vi "main.vi"(1 "chessboard_size":u8=8, 2 "starting_square":T1) -> ()   [LabVIEW 2020, in "core.lvlib"]
uses:
  core.lvlib
  core_data/chess_square--chess notation.ctl
  core_data/file--enum.ctl
  core_data/rank--enum.ctl
  action.ctl
  check_has_tour_been_found.vi
  check_has_unreacheable_square_been_formed.vi
  check_any_corner_islands.vi
  convert--duration to formatted string.vi
  get_chessboard_square.vi
  check_island.vi
  check_head_is_neighbour.vi
  get all unexplored neighbours.vi
  pause (global variable).vi
  core_data/library_variable.vi
  pause after every move (global variable).vi
  main/Enqueue--button_press_pause.vi
  core_wait (global variable).vi
  convert--chessboard_index to chess_square (string).vi
  get tour type.vi
  core_data/chessboard_index.ctl
  core_data/completed_tour.ctl
  core_data/tour type (enum).ctl
  core_data/core_data.lvlib
  core_data/tour_in_progress.ctl
  core_data/core_data.ctl
  core_data/neighbour_square.ctl
  core_data/chess_square.ctl
  global_stop_flag/global_stop_flag.lvlib
  main/main.lvlib
  PTRL/timing_utilities/timing_utilities.lvlib
  PTRL/dev_and_debug_tools/dev_and_debug_tools.lvlib
panel:
  out "complete_tour indexes":i32[](array[numeric])
  out "States out (index 0 = oldest)":string[](array[string])
  out "iteration":i32
  # "Core"
  # "Development\ncontrols/indicators useful for development and testing, but which are not outputs of the VI"
  # "Input\nInputs to the VI"
  # "Output\nOutputs of the VI"
  # "Description\n\nBlank VI with error handling case. \n\nSummarize the use of this VI in this space."
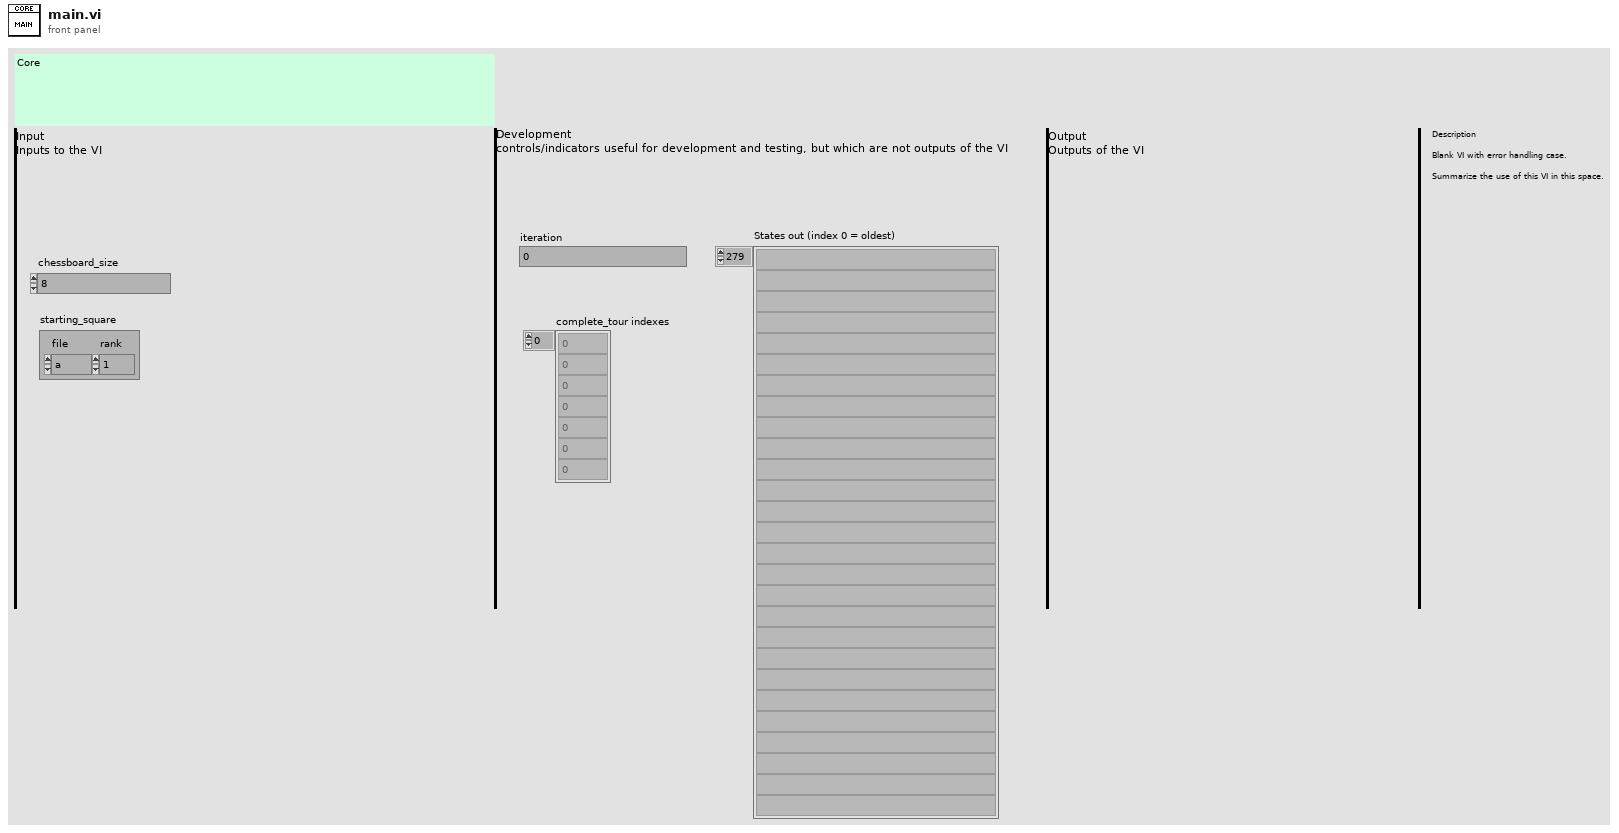
[diagram p1: front panel]
types:
  T1 = typedef "core.lvlib/core_data.lvlib/chess_square--chess notation.ctl" = cluster{"file":T2, "rank":T3}
  T2 = typedef "core.lvlib/core_data.lvlib/file--enum.ctl" = enum16{"a", "b", "c", "d", "e", "f", "g", "h"}
  T3 = typedef "core.lvlib/core_data.lvlib/rank--enum.ctl" = enum16{"1", "2", "3", "4", "5", "6", "7", "8"}
  T4 = typedef "core.lvlib/action.ctl" = enum16{"init", "move_forward", "move_backward", "complete_tour", "exit", "be idle (do nothing)"}
  T5 = typedef "core.lvlib/core_data.lvlib/chessboard_index.ctl" = cluster{"row":u8, "column":u8}
  T6 = typedef "core.lvlib/core_data.lvlib/core_data.ctl" = cluster{"tour_in_progress":T7, "total no. of moves forward":u64, "total no. of moves backward":u64, "chessboard":T8[][], "square_to_move_forward_to":T5}
  T7 = typedef "core.lvlib/core_data.lvlib/tour_in_progress.ctl" = cluster{"start_time":timestamp, "tour":T5[], "no. of moves forward":u64, "no. of moves backward":u64}
  T8 = typedef "core.lvlib/core_data.lvlib/chess_square.ctl" = cluster{"Explored?":bool, "neighbouring_squares":T9[]}
  T9 = typedef "core.lvlib/core_data.lvlib/neighbour_square.ctl" = cluster{"row":u8, "column":u8, "exhausted?":bool}
  T10 = typedef "core.lvlib/core_data.lvlib/completed_tour.ctl" = cluster{"complete_tour":T5[], "start square":string, "end square":string, "tour type":T11, "start_time":timestamp, "end_time":timestamp, "duration (seconds)":dbl, "duration (formatted string)":string, "no. of moves forward":u64, "no. of moves backward":u64, "total no. of moves since core started running":u64}
  T11 = typedef "core.lvlib/core_data.lvlib/tour type (enum).ctl" = enum16{"open", "closed"}
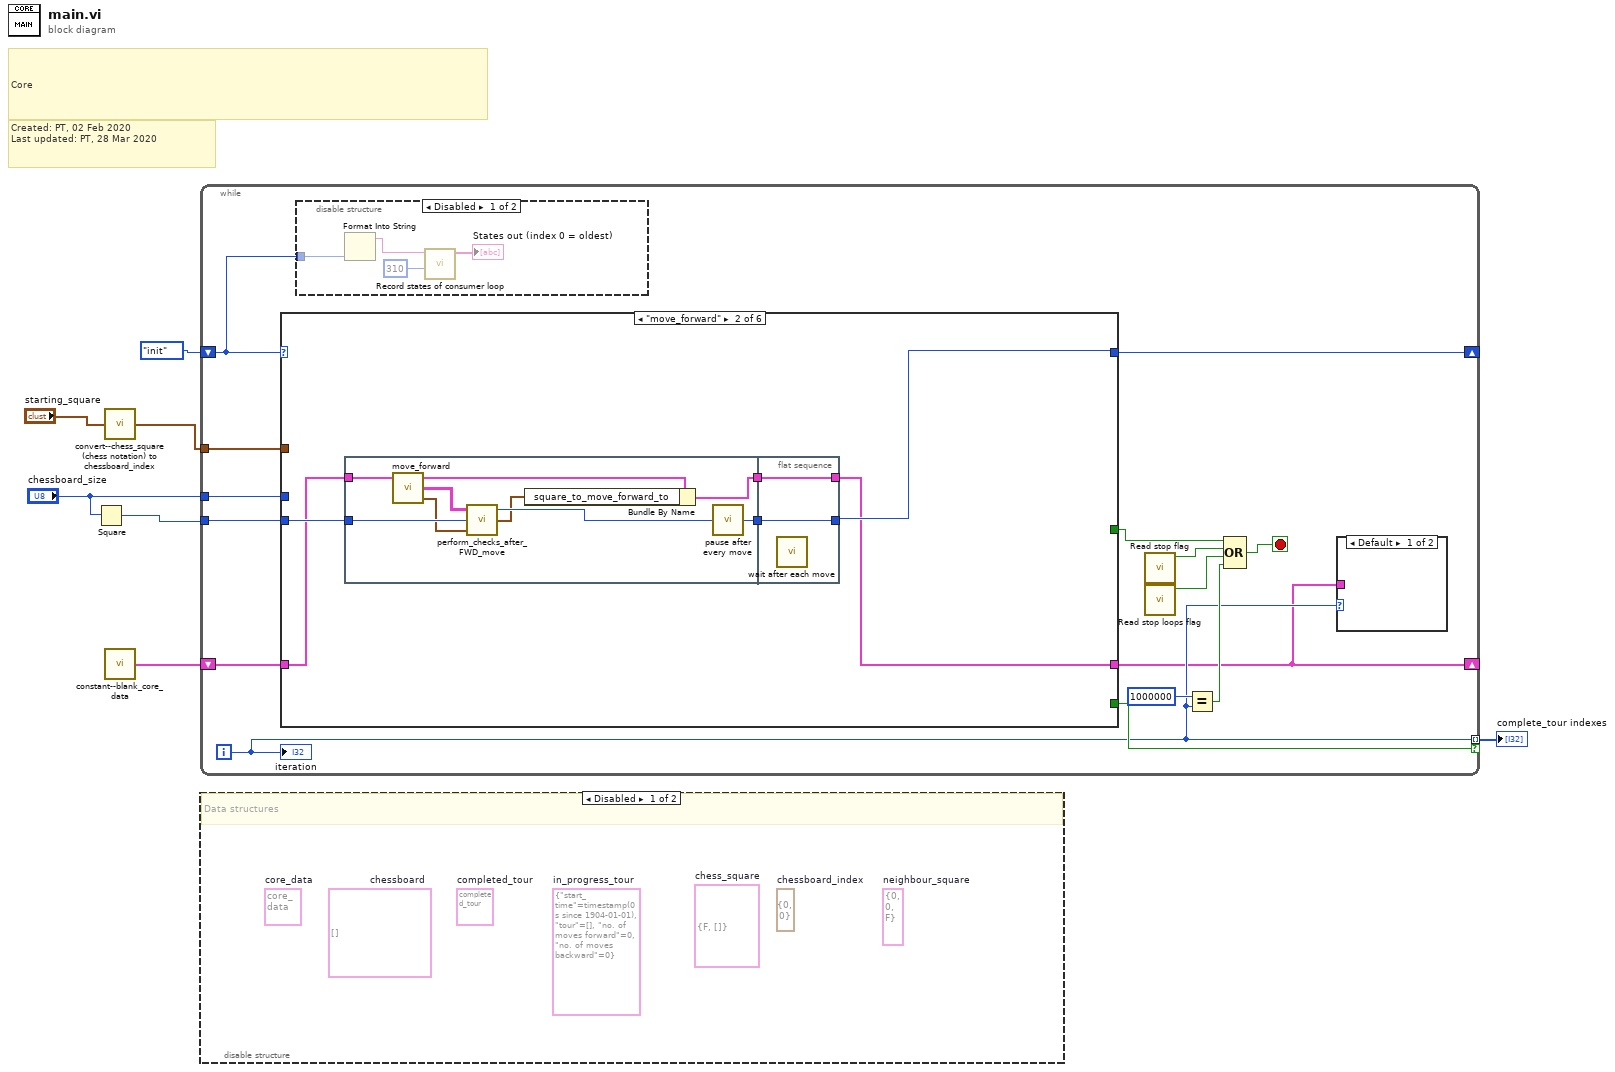
[diagram p0: block diagram]
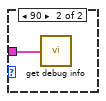
[diagram p3: hidden frame]
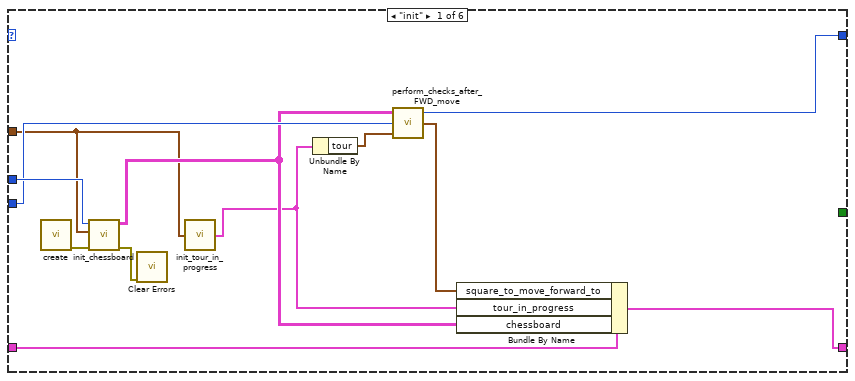
[diagram p4: hidden frame]
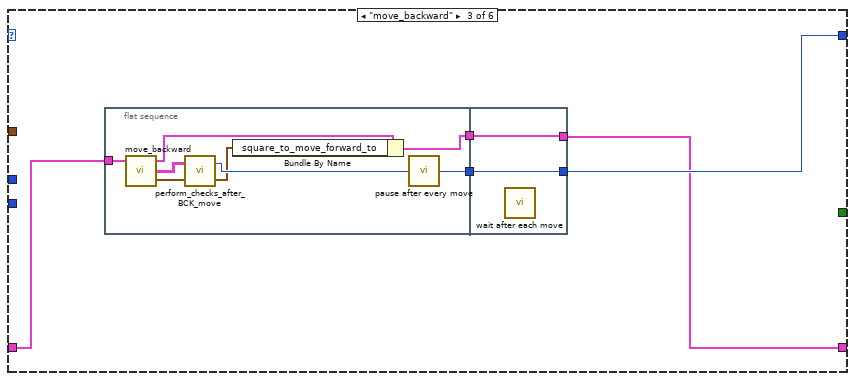
[diagram p5: hidden frame]
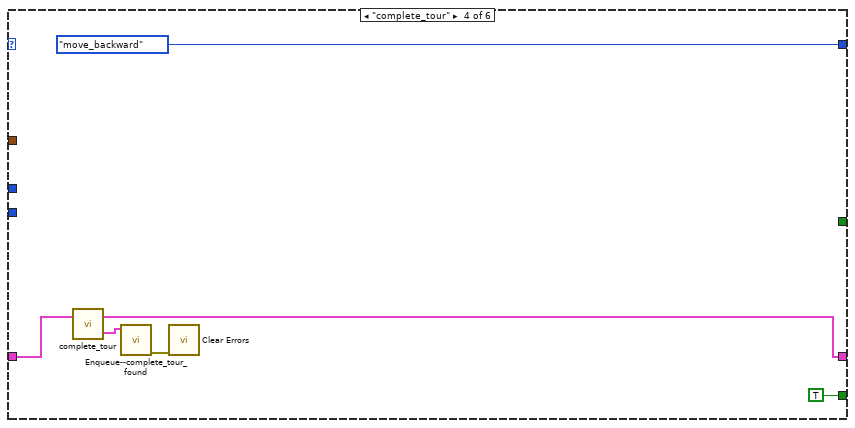
[diagram p6: hidden frame]
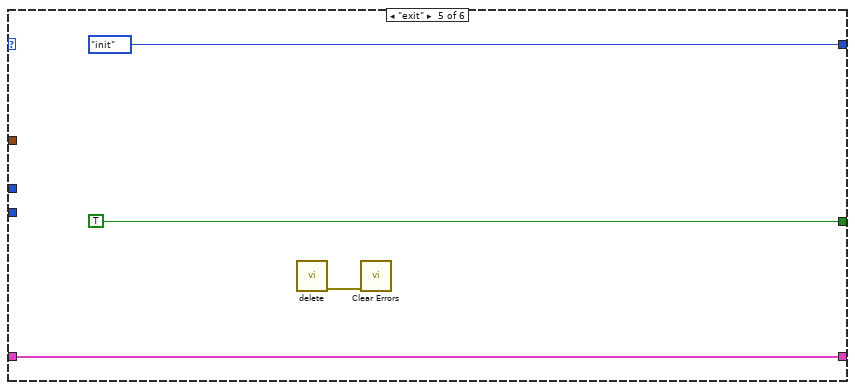
[diagram p7: hidden frame]
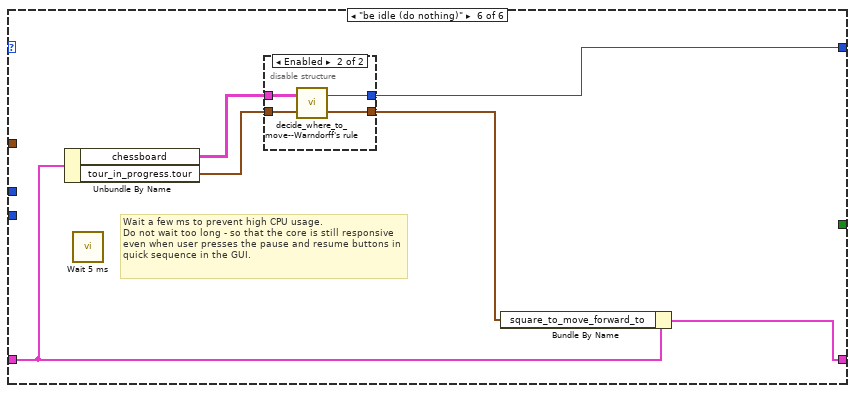
[diagram p8: hidden frame]
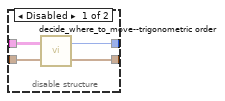
[diagram p9: hidden frame]
diagram:
  # "Core"
  # "Created: PT, 02 Feb 2020\nLast updated: PT, 28 Mar 2020"
  n1 = Square(x="chessboard_size") -> (x^2=w5:u8)
  n2 = call "convert--chess_square (chess notation) to chessboard_index.vi"("chess_square (chess notation)"="starting_square") -> ("chessboard_index"=w3:T5)
  n3 = call "constant--blank_core_data.vi"() -> ("blank core_data"=w2:T6)
  n4 = while {
    shift-right: [w22] -> _
    shift-left: action."init" ("action (default = init)") -> [w13]
    tunnel: w3 -> [w21]
    tunnel: "chessboard_size" -> [w20]
    tunnel: w5 -> [w15]
    shift-right: [w8] -> _
    shift-left: w2 -> [w14]
    tunnel: [w9] -> w1 mode=indexing if=w10
    i -> [w9]
    stop <- w18 stop-if-true
    n5 = case shown="\"move_forward\"" w13 {
      tunnel: [w36 w45 w60 action."move_backward" ("action") action."init" ("action") w87] -> w22
      tunnel: w21 -> [w34 _ _ _ _ _]
      tunnel: w20 -> [w39 _ _ _ _ _]
      tunnel: w15 -> [w37 w43 _ _ _ _]
      tunnel: [_ _ _ _ TRUE _] -> w19
      tunnel: w14 -> [w32 w42 w59 w74 w79 w83]
      tunnel: [w30 w40 w57 w73 w79 w84] -> w8
      tunnel: [_ _ _ TRUE _ _] -> w10
      frame "init" {
        n6 = call "create.vi"() -> ("error out"=w38:errorcluster)  [unwired: 11 in]
        n7 = call "init_chessboard.vi"("error in (no error)"=w38, "starting_square"=w34, "chessboard_size"=w39) -> ("error out"=w33:errorcluster, "chessboard (populated)"=w35:T8[][])  [unwired: 7 in]
        n8 = call <vilib>:"Clear Errors.vi"("error in (no error)"=w33) -> ()  [unwired: 5 in, 2 out]
        n9 = call "init_tour_in_progress.vi"("starting_square"=w34) -> ("blank_tour_in_progress"=w28:T7)
        n10 = Unbundle By Name(w28) -> ("tour"=w31:T5[])
        n11 = call "perform_checks_after_FWD_move.vi"("tour_in_progress"=w31, "no. of squares on chessboard"=w37, "chessboard"=w35) -> ("square_to_move_forward_to"=w29:T5, "next action"=w36:T4)  [unwired: 1 in]
        n12 = Bundle By Name(cluster=w32, "square_to_move_forward_to"=w29, "tour_in_progress"=w28, "chessboard"=w35) -> (w30:T6)
      }
      frame "move_forward" {
        n13 = flat-sequence {
          tunnel: [w53] -> w44
          tunnel: w43 -> [w51]
          tunnel: w42 -> [w49]
          tunnel: [w47] -> w41
          tunnel: [w56] -> w45
          tunnel: w44 -> [w56]
          tunnel: [w55] -> w40
          tunnel: w41 -> [w55]
          frame #0 {
            n14 = call "move_forward.vi"("core_data in"=w49) -> ("tour in progress"=w50:T5[], "chessboard"=w52:T8[][], "core_data out"=w48:T6)  [unwired: 2 in]
            n15 = call "perform_checks_after_FWD_move.vi"("tour_in_progress"=w50, "no. of squares on chessboard"=w51, "chessboard"=w52) -> ("square_to_move_forward_to"=w46:T5, "next action"=w54:T4)  [unwired: 1 in]
            n16 = Bundle By Name(cluster=w48, "square_to_move_forward_to"=w46) -> (w47:T6)
            n17 = call "pause after every move.vi"("next action in"=w54) -> ("next action out"=w53:T4)
          }
          frame #1 {
            n18 = call "wait after each move.vi"() -> ()  [unwired: 12 in]
          }
        }
      }
      frame "move_backward" {
        n19 = flat-sequence {
          tunnel: [w68] -> w61
          tunnel: w59 -> [w65]
          tunnel: [w63] -> w58
          tunnel: [w71] -> w60
          tunnel: w61 -> [w71]
          tunnel: [w70] -> w57
          tunnel: w58 -> [w70]
          frame #0 {
            n20 = call "move_backward.vi"("core_data in"=w65) -> ("tour in progress"=w66:T5[], "chessboard"=w67:T8[][], "core_data out"=w64:T6)  [unwired: 2 in]
            n21 = call "perform_checks_after_BCK_move.vi"("tour in progress"=w66, "chessboard"=w67) -> ("square_to_move_forward_to"=w62:T5, "next action"=w69:T4)
            n22 = Bundle By Name(cluster=w64, "square_to_move_forward_to"=w62) -> (w63:T6)
            n23 = call "pause after every move.vi"("next action in"=w69) -> ("next action out"=w68:T4)
          }
          frame #1 {
            n24 = call "wait after each move.vi"() -> ()  [unwired: 12 in]
          }
        }
      }
      frame "complete_tour" {
        n25 = call "complete_tour.vi"("core_data in"=w74) -> ("the recently completed tour"=w75:T10, "core_data out"=w73:T6)  [unwired: 1 in]
        n26 = call "Enqueue--complete_tour_found.vi"("completed_tour"=w75) -> ("error out"=w76:errorcluster)  [unwired: 10 in]
        n27 = call <vilib>:"Clear Errors.vi"("error in (no error)"=w76) -> ()  [unwired: 5 in, 2 out]
      }
      frame "exit" {
        n28 = call "delete.vi"() -> ("error out"=w78:errorcluster)  [unwired: 10 in, 1 out]
        n29 = call <vilib>:"Clear Errors.vi"("error in (no error)"=w78) -> ()  [unwired: 5 in, 2 out]
      }
      frame "be idle (do nothing)" {
        # "Wait a few ms to prevent high CPU usage.\nDo not wait too long - so that the core is still responsive even when user presses the pause and resume buttons in quick sequence in the GUI."
        n30 = Unbundle By Name(w83) -> ("chessboard"=w86:T8[][], "tour_in_progress.tour"=w85:T5[])
        n31 = call "Wait 5 ms.vi"() -> ()  [unwired: 11 in, 1 out]
        n32 = disable-structure shown="Enabled" {
          disable-tunnel: [w91 w92] -> w82
          disable-tunnel: [w90 w93] -> w87
          disable-tunnel: w86 -> [w89 w95]
          disable-tunnel: w85 -> [w88 w94]
          frame Disabled {
            n33 = call "decide_where_to_move--trigonometric order.vi"("tour_in_progress"=w88, "chessboard"=w89) -> ("square_to_move_forward_to"=w91:T5, "action"=w90:T4)
          }
          frame Enabled {
            n34 = call "decide_where_to_move--Warndorff's rule.vi"("tour_in_progress"=w94, "chessboard"=w95) -> ("square_to_move_forward_to"=w92:T5, "action"=w93:T4)
          }
        }
        n35 = Bundle By Name(cluster=w83, "square_to_move_forward_to"=w82) -> (w84:T6)
      }
    }
    n36 = disable-structure shown="Disabled" {
      disable-tunnel: w13 -> [w26 _]
      frame Disabled {
        n37 = Format Into String(w26) -> (resulting string=w25:string)  [unwired: 3 in, 1 out]
        n38 = call "Record states of consumer loop.vi"("n (dflt=100)"=u32 310, "State in"=w25) -> ("States out (index 0 = oldest)"=→"States out (index 0 = oldest)":string[])  [unwired: 7 in, 2 out]
      }
      frame Enabled {
      }
    }
    n39 = call "Read stop flag.vi"() -> ("Stop core?"=w17:bool)  [unwired: 10 in, 1 out]
    n40 = call "Read stop loops flag.vi"() -> ("Stop all loops?"=w16:bool)  [unwired: 10 in, 1 out]
    n41 = Equal?(x=1000000, y=w9) -> (x = y?=w12:bool)
    n42 = Compound Arithmetic op=OR(w19, w17, w16, w12) -> (w18:bool)
    n43 = case shown="Default" w9 {
      tunnel: w8 -> [_ w27]
      frame Default {
      }
      frame 90 {
        n44 = call "get debug info.vi"("core_data"=w27) -> ()
      }
    }
    "iteration" <- w9
  }
  "complete_tour indexes" <- w1
  n45 = disable-structure shown="Disabled" {
    frame Disabled {
      (unwired) T8[][] []  # chessboard
      (unwired) T9 {"row"=0, "column"=0, "exhausted?"=FALSE}  # neighbour_square
      (unwired) T10 {"complete_tour"=[], "start square"="", "end square"="", "tour type"=enum."open", "start_time"=timestamp(0 s since 1904-01-01), "end_time"=timestamp(0 s since 1904-01-01), "duration (seconds)"=0.0, "duration (formatted string)"="", "no. of moves forward"=0, "no. of moves backward"=0, "total no. of moves since core started running"=0}  # completed_tour
      (unwired) T5 {"row"=0, "column"=0}  # chessboard_index
      (unwired) T8 {"Explored?"=FALSE, "neighbouring_squares"=[]}  # chess_square
      (unwired) T7 {"start_time"=timestamp(0 s since 1904-01-01), "tour"=[], "no. of moves forward"=0, "no. of moves backward"=0}  # in_progress_tour
      (unwired) T6 {"tour_in_progress"={"start_time"=timestamp(0 s since 1904-01-01), "tour"=[], "no. of moves forward"=0, "no. of moves backward"=0}, "total no. of moves forward"=0, "total no. of moves backward"=0, "chessboard"=[], "square_to_move_forward_to"={"row"=0, "column"=0}}  # core_data
      # "Data structures"
    }
    frame Enabled {
    }
  }
